vi "Ejercicio 3.3.vi"() -> ()   [LabVIEW 2021]
panel:
  out "Waveform Graph 3":dbl[](graph)
  out "Waveform Graph 2":dbl[](graph)
  out "Waveform Graph 1":dbl[](graph)
  out "fila 3":dbl[](array[numeric])
  out "fila 2":dbl[](array[numeric])
  out "fila 1":dbl[](array[numeric])
  out "Array":dbl[][](array[numeric])
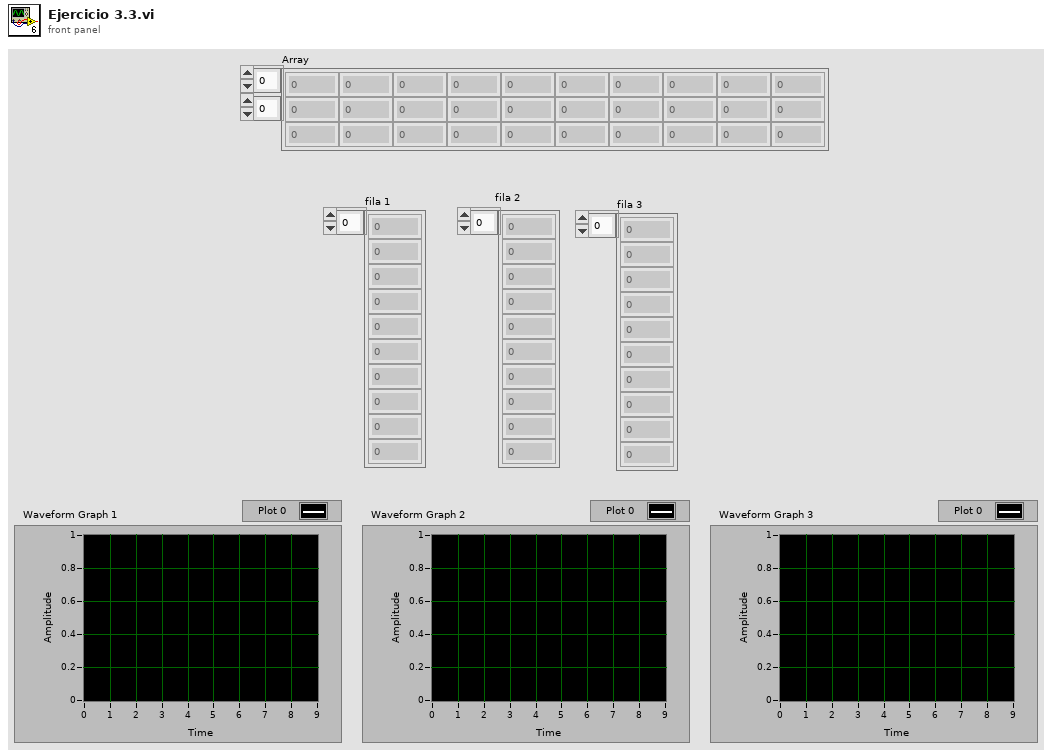
[diagram p1: front panel]
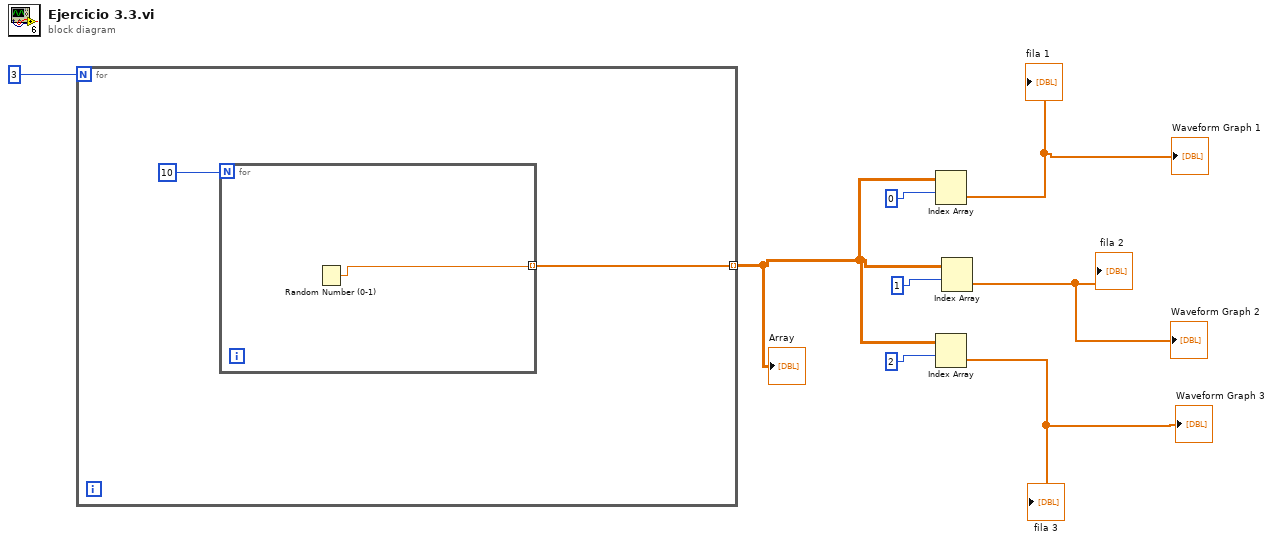
[diagram p0: block diagram]
diagram:
  n1 = for {
    N: 3 -> [_]
    tunnel: [w9] -> w4 mode=indexing
    n2 = for {
      N: 10 -> [_]
      tunnel: [w11] -> w9 mode=indexing
      n3 = Random Number (0-1)() -> (number: 0 to 1=w11:dbl)
    }
  }
  "Array" <- w4
  n4 = Index Array(array=w4, index (row)=0) -> (element=→"fila 1" →"Waveform Graph 1":dbl[])  [unwired: 1 in]
  n5 = Index Array(array=w4, index (row)=2) -> (element=→"fila 3" →"Waveform Graph 3":dbl[])  [unwired: 1 in]
  n6 = Index Array(array=w4, index (row)=1) -> (element=→"fila 2" →"Waveform Graph 2":dbl[])  [unwired: 1 in]
